vi "configure.vi"(8 "error in (no error)":errorcluster, 9 "Value":i32, 10 "ILC":refnum<class "ILC.lvclass">, 11 "ConfigureILCSSRStrategy in":refnum<class "ConfigureILCDCAPressureStrategy.lvclass">) -> (0 "error out":errorcluster, 2 "ILC 2":refnum<class "ILC.lvclass">, 3 "ConfigureILCSSRStrategy out":refnum<class "ConfigureILCDCAPressureStrategy.lvclass">)   [LabVIEW 2015, in "ConfigureILCDCAPressureStrategy.lvclass"]
uses:
  ConfigureILCDCAPressureStrategy.lvclass
  <userlib>/Common/ILC/ILC/ILC.lvclass
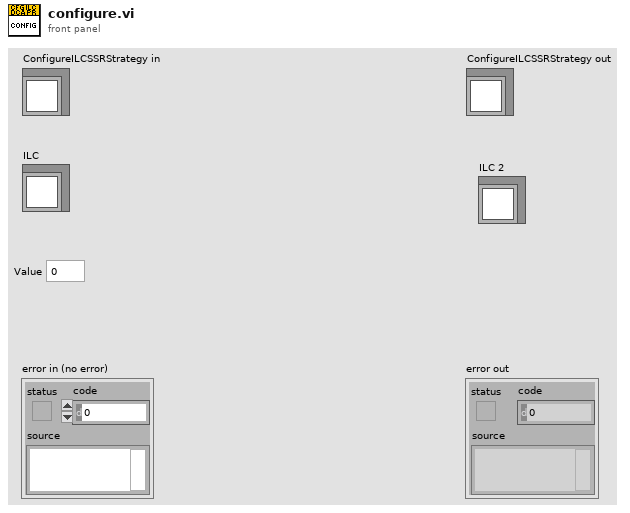
[diagram p1: front panel]
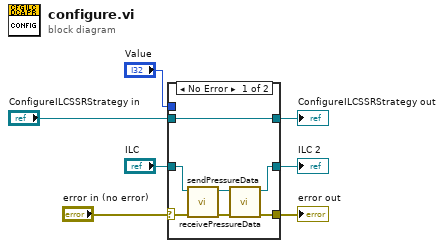
[diagram p0: block diagram]
diagram:
  n1 = case shown="No Error" "error in (no error)" {
    selector: "error in (no error)" -> [w12 w17]
    tunnel: [w9 w17] -> w6
    tunnel: [w14 w16] -> w4
    tunnel: "ConfigureILCSSRStrategy in" -> [w14 w16]
    tunnel: "ILC" -> [w13 w15]
    tunnel: "Value" -> [_ _]
    tunnel: [w8 w15] -> w1
    frame No Error {
      n2 = call <userlib>:"sendPressureData.vi"("error in (no error)"=w12, "ILC in"=w13) -> ("error out"=w10:errorcluster, "ILC out"=w11:refnum<class "ILC.lvclass">)  [unwired: 8 in]
      n3 = call <userlib>:"receivePressureData.vi"("error in (no error)"=w10, "ILC in"=w11) -> ("error out"=w9:errorcluster, "ILC out"=w8:refnum<class "ILC.lvclass">)  [unwired: 8 in]
    }
    frame Error {
    }
  }
  "error out" <- w6
  "ConfigureILCSSRStrategy out" <- w4
  "ILC 2" <- w1
